vi "Gather Relevant Data.vi"(11 "Sorted Data":dbl[][](array[numeric])) -> (3 "Relevant Data":T1(array[cluster]))   [LabVIEW 2015]
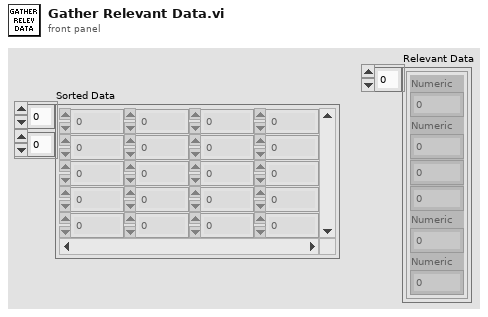
[diagram p1: front panel]
types:
  T1 = cluster{"Numeric":dbl, "Numeric":dbl, dbl, dbl, "Numeric":dbl, "Numeric":dbl}[]
  T2 = cluster{"Numeric":dbl, "Numeric":dbl, dbl, dbl, "Numeric":dbl, "Numeric":dbl}
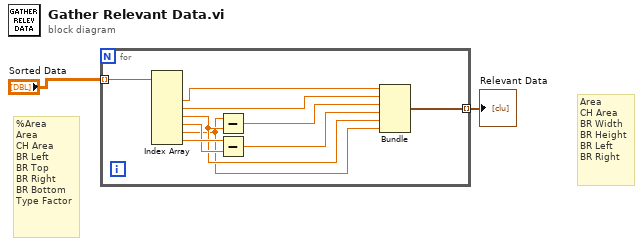
[diagram p0: block diagram]
diagram:
  # "Area\nCH Area\nBR Width\nBR Height\nBR Left\nBR Right"
  # "%Area\nArea\nCH Area\nBR Left\nBR Top\nBR Right\nBR Bottom\nType Factor"
  n1 = for {
    tunnel: "Sorted Data" -> [w10] mode=indexing
    tunnel: [w5] -> w1 mode=indexing
    n2 = Index Array(array=w10) -> (element #2=w12:dbl, element #3=w11:dbl, element #4=w4:dbl, element #5=w8:dbl, element #6=w3:dbl, element #7=w9:dbl)  [unwired: 7 in, 1 out]
    n3 = Subtract(x=w3, y=w4) -> (x-y=w7:dbl)
    n4 = Subtract(x=w9, y=w8) -> (x-y=w6:dbl)
    n5 = Bundle("Numeric"=w12, "Numeric"=w11, w7, w6, "Numeric"=w4, "Numeric"=w3) -> (w5:T2)  [unwired: 1 in]
  }
  "Relevant Data" <- w1
